vi "one matrix 1-14 graph.vi"(1 "dt":dbl, 2 "Applica filtro 4":u16, 3 "Dati 2":dbl[][](array[numeric])) -> (0 "Waveform Graph":waveform(dbl)[](graph))   [LabVIEW 2012]
uses:
  <vilib>/Analysis/NI_AALBase.lvlib
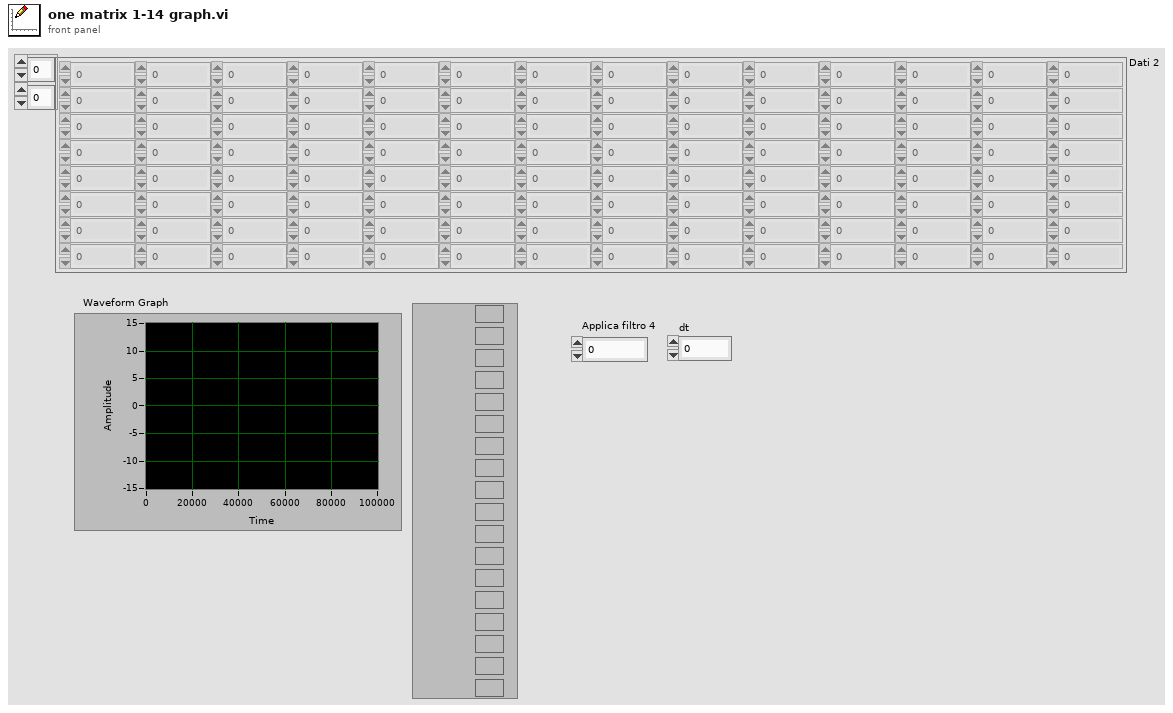
[diagram p1: front panel]
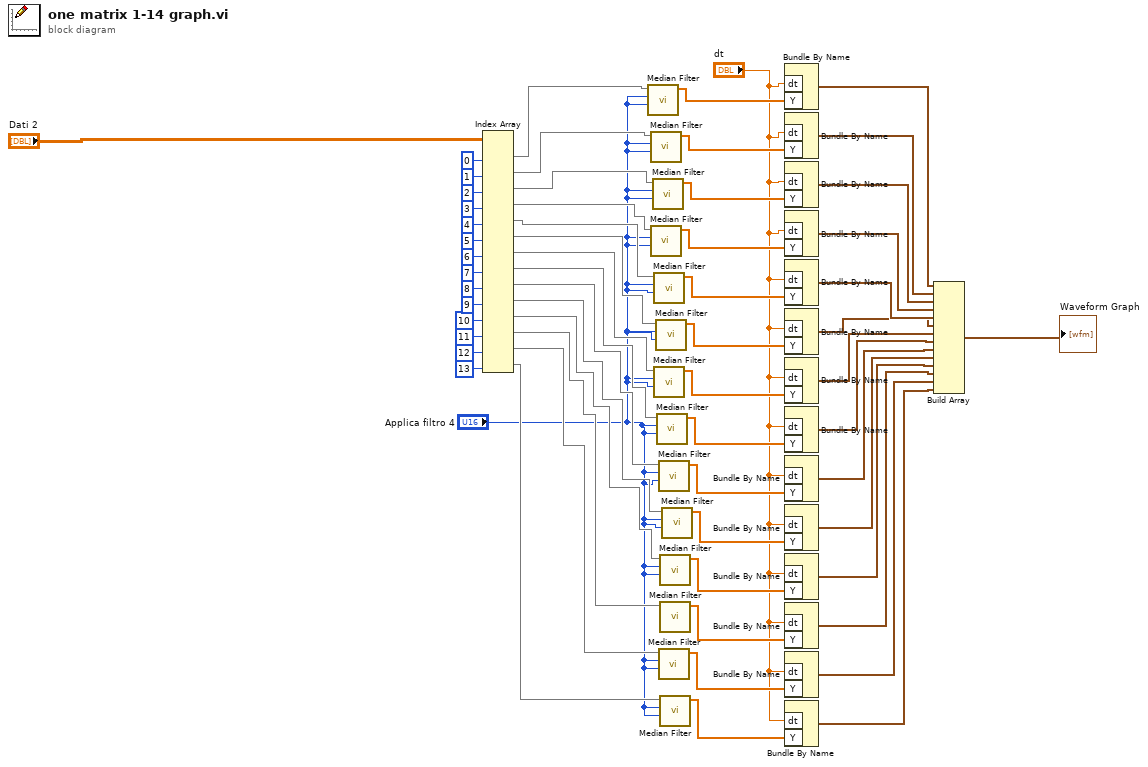
[diagram p0: block diagram]
diagram:
  n1 = Index Array(array="Dati 2", index (col) #1=0 ("disabled index (col)"), index (col) #2=1 ("index (col)"), index (col) #3=2 ("index (col)"), index (col) #4=3 ("index (col)"), index (col) #5=4 ("index (col)"), index (col) #6=5 ("index (col)"), index (col) #7=6 ("index (col)"), index (col) #8=7 ("index (col)"), index (col) #9=8 ("index (col)"), index (col) #10=9 ("index (col)"), index (col) #11=10 ("index (col)"), index (col) #12=11 ("index (col)"), index (col) #13=12 ("index (col)"), index (col) #14=13 ("index (col)")) -> (element #1=w45:dbl[], element #2=w44:dbl[], element #3=w43:dbl[], element #4=w42:dbl[], element #5=w41:dbl[], element #6=w40:dbl[], element #7=w39:dbl[], element #8=w38:dbl[], element #9=w37:dbl[], element #10=w36:dbl[], element #11=w35:dbl[], element #12=w34:dbl[], element #13=w33:dbl[], element #14=w32:dbl[])  [unwired: 14 in]
  n2 = call <vilib>:"Median Filter.vi"("right rank"="Applica filtro 4", "left rank"="Applica filtro 4", "X"=w45) -> ("Filtered X"=w30:dbl[])  [unwired: 7 in, 1 out]
  n3 = call <vilib>:"Median Filter.vi"("right rank"="Applica filtro 4", "left rank"="Applica filtro 4", "X"=w44) -> ("Filtered X"=w29:dbl[])  [unwired: 7 in, 1 out]
  n4 = call <vilib>:"Median Filter.vi"("right rank"="Applica filtro 4", "left rank"="Applica filtro 4", "X"=w42) -> ("Filtered X"=w27:dbl[])  [unwired: 7 in, 1 out]
  n5 = call <vilib>:"Median Filter.vi"("right rank"="Applica filtro 4", "left rank"="Applica filtro 4", "X"=w43) -> ("Filtered X"=w28:dbl[])  [unwired: 7 in, 1 out]
  n6 = call <vilib>:"Median Filter.vi"("right rank"="Applica filtro 4", "left rank"="Applica filtro 4", "X"=w41) -> ("Filtered X"=w26:dbl[])  [unwired: 7 in, 1 out]
  n7 = call <vilib>:"Median Filter.vi"("right rank"="Applica filtro 4", "left rank"="Applica filtro 4", "X"=w39) -> ("Filtered X"=w24:dbl[])  [unwired: 7 in, 1 out]
  n8 = call <vilib>:"Median Filter.vi"("right rank"="Applica filtro 4", "left rank"="Applica filtro 4", "X"=w40) -> ("Filtered X"=w25:dbl[])  [unwired: 7 in, 1 out]
  n9 = call <vilib>:"Median Filter.vi"("right rank"="Applica filtro 4", "left rank"="Applica filtro 4", "X"=w38) -> ("Filtered X"=w23:dbl[])  [unwired: 7 in, 1 out]
  n10 = call <vilib>:"Median Filter.vi"("right rank"="Applica filtro 4", "left rank"="Applica filtro 4", "X"=w37) -> ("Filtered X"=w22:dbl[])  [unwired: 7 in, 1 out]
  n11 = call <vilib>:"Median Filter.vi"("right rank"="Applica filtro 4", "left rank"="Applica filtro 4", "X"=w33) -> ("Filtered X"=w18:dbl[])  [unwired: 7 in, 1 out]
  n12 = call <vilib>:"Median Filter.vi"("right rank"="Applica filtro 4", "left rank"="Applica filtro 4", "X"=w35) -> ("Filtered X"=w20:dbl[])  [unwired: 7 in, 1 out]
  n13 = call <vilib>:"Median Filter.vi"("X"=w34) -> ("Filtered X"=w19:dbl[])  [unwired: 9 in, 1 out]
  n14 = call <vilib>:"Median Filter.vi"("right rank"="Applica filtro 4", "left rank"="Applica filtro 4", "X"=w32) -> ("Filtered X"=w17:dbl[])  [unwired: 7 in, 1 out]
  n15 = call <vilib>:"Median Filter.vi"("right rank"="Applica filtro 4", "left rank"="Applica filtro 4", "X"=w36) -> ("Filtered X"=w21:dbl[])  [unwired: 7 in, 1 out]
  n16 = Bundle By Name("dt"="dt", "Y"=w30) -> (w16:waveform(dbl))  [unwired: 1 in]
  n17 = Bundle By Name("dt"="dt", "Y"=w29) -> (w15:waveform(dbl))  [unwired: 1 in]
  n18 = Bundle By Name("dt"="dt", "Y"=w28) -> (w14:waveform(dbl))  [unwired: 1 in]
  n19 = Bundle By Name("dt"="dt", "Y"=w27) -> (w13:waveform(dbl))  [unwired: 1 in]
  n20 = Bundle By Name("dt"="dt", "Y"=w26) -> (w12:waveform(dbl))  [unwired: 1 in]
  n21 = Bundle By Name("dt"="dt", "Y"=w25) -> (w11:waveform(dbl))  [unwired: 1 in]
  n22 = Bundle By Name("dt"="dt", "Y"=w24) -> (w10:waveform(dbl))  [unwired: 1 in]
  n23 = Bundle By Name("dt"="dt", "Y"=w23) -> (w9:waveform(dbl))  [unwired: 1 in]
  n24 = Bundle By Name("dt"="dt", "Y"=w22) -> (w8:waveform(dbl))  [unwired: 1 in]
  n25 = Bundle By Name("dt"="dt", "Y"=w21) -> (w7:waveform(dbl))  [unwired: 1 in]
  n26 = Bundle By Name("dt"="dt", "Y"=w20) -> (w6:waveform(dbl))  [unwired: 1 in]
  n27 = Bundle By Name("dt"="dt", "Y"=w19) -> (w5:waveform(dbl))  [unwired: 1 in]
  n28 = Bundle By Name("dt"="dt", "Y"=w18) -> (w4:waveform(dbl))  [unwired: 1 in]
  n29 = Bundle By Name("dt"="dt", "Y"=w17) -> (w3:waveform(dbl))  [unwired: 1 in]
  n30 = Build Array(w16, w15, w14, w13, w12, w11, w10, w9, w8, w7, w6, w5, w4, w3) -> (→"Waveform Graph":waveform(dbl)[])
